vi "GWInstek  GDM8351 Acquire Multiple.vi"() -> ()   [LabVIEW 2021]
doc: "This example shows how to configure a measurement and take multiple readings."
uses:
  <instrlib>/GWInstek  GDM8351/Public/Data/Read (Multiple Points).vi
  <instrlib>/GWInstek  GDM8351/GWInstek  GDM8351.lvlib
panel:
  in  "Baud Rate (115200)":u32(ring)=115200 items=["9600"=9600, "19200"=19200, "38400"=38400, "57600"=57600, "115200"=115200]
  in  "Function (0: DC Volts)":i32(ring) items=["DC Volts", "AC Volts", "DC+AC Volts", "DC Current", "AC Current", "DC+AC Current", "2-Wire Resistance", "4-Wire Resistance", "Frequency", "Period", "Continuity", "Diode", "Temperature", "Capacitance"]
  in  "Sample Count (1)":i32=1 format="%#.6g"
  out "Measurements":dbl[](array[numeric])
  in  "Timeout (10000 ms)":i32=10000 format="%#.6g"
  in  "VISA resource name":refnum<visa-resource-name>
  # "(c) 2014 GWInstek.  ALL RIGHTS RESERVED."
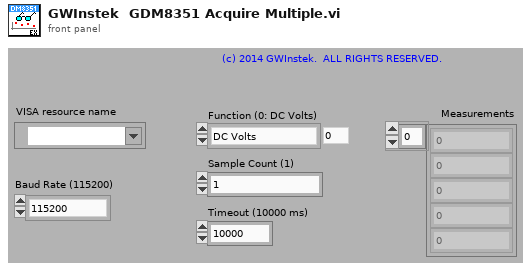
[diagram p1: front panel]
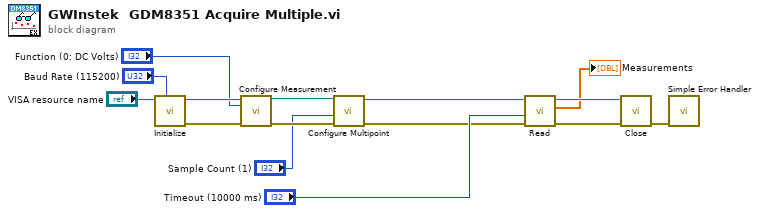
[diagram p0: block diagram]
diagram:
  n1 = call <instrlib>:"Initialize.vi"("Baud Rate (115200)"="Baud Rate (115200)", "VISA resource name"="VISA resource name") -> ("error out"=w12:errorcluster, "VISA resource name out"=w13:refnum<visa-resource-name>)  [unwired: 8 in]
  n2 = call <instrlib>:"Configure Measurement.vi"("VISA resource name"=w13, "Function (0: DC Volts)"="Function (0: DC Volts)", "error in (no error)"=w12) -> ("VISA resource name out"=w8:refnum<visa-resource-name>, "error out"=w5:errorcluster)  [unwired: 11 in]
  n3 = call <instrlib>:"Configure Multipoint.vi"("error in (no error)"=w5, "Sample Count (1)"="Sample Count (1)", "VISA resource name"=w8) -> ("error out"=w4:errorcluster, "VISA resource name out"=w6:refnum<visa-resource-name>)  [unwired: 7 in]
  n4 = call-poly <instrlib>:"Read.vi"("error in (no error)"=w4, "Timeout (10000 ms)"="Timeout (10000 ms)", "VISA resource name"=w6) -> ("error out"=w11:errorcluster, "Measurements"=→"Measurements":dbl[], "VISA resource name out"=w10:refnum<visa-resource-name>)  [unwired: 6 in]
  n5 = call <instrlib>:"Close.vi"("error in (no error)"=w11, "VISA resource name"=w10) -> ("error out"=w15:errorcluster)  [unwired: 9 in]
  n6 = call <vilib>:"Simple Error Handler.vi"("error in (no error)"=w15) -> ()  [unwired: 4 in, 5 out]
